vi "Create Config File Header.vi"(8 "error in (no error)":errorcluster, 10 "Path":path, 11 "Config Parser BML in":refnum<class "Config Parser BML.lvclass">) -> (0 "error out":errorcluster, 3 "Config Parser BML out":refnum<class "Config Parser BML.lvclass">)   [LabVIEW 2018, in "Config Parser BML.lvlib" / "Config Parser BML.lvclass"]
uses:
  Config Parser BML.lvclass
  <vilib>/Utility/file.llb/Write Delimited Spreadsheet (string).vi
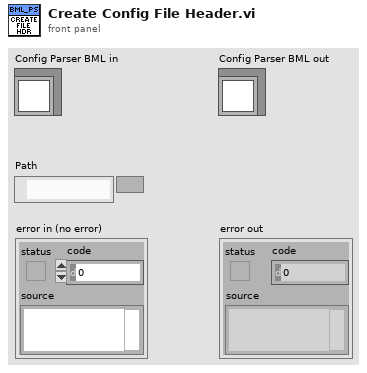
[diagram p1: front panel]
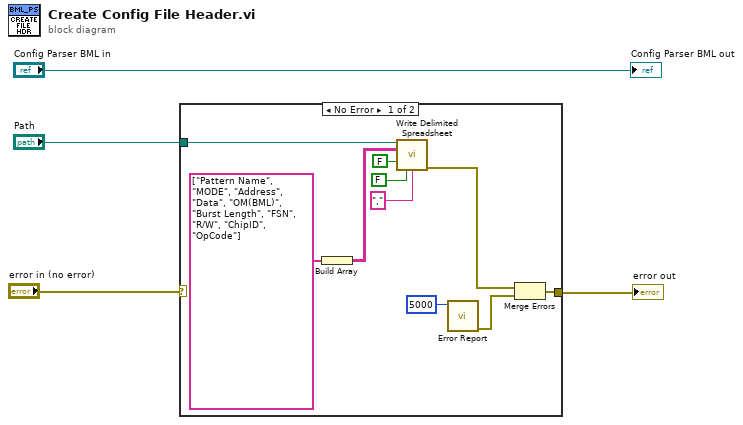
[diagram p0: block diagram]
diagram:
  n1 = case shown="No Error" "error in (no error)" {
    selector: "error in (no error)" -> [_ w15]
    tunnel: "Path" -> [w12 _]
    tunnel: [w7 w15] -> w1
    frame No Error {
      n2 = Build Array(string[] ["Pattern Name", "MODE", "Address", "Data", "OM(BML)", "Burst Length", "FSN", "R/W", "ChipID", "OpCode"]) -> (w10:string[][])
      n3 = call-poly <vilib>:"Write Delimited Spreadsheet.vi"("file path (dialog if empty)"=w12, "2D data"=w10, "append to file? (new file:F)"=FALSE, "transpose? (no:F)"=FALSE, "delimiter (\\t)"="," ("delimiter (\\t)")) -> ("error out"=w6:errorcluster)  [unwired: 9 in, 1 out]
      n4 = call "Error Report.vi"("Error Code"=i16 5000) -> ("error out"=w5:errorcluster)  [unwired: 10 in]
      n5 = Merge Errors(w6, w5) -> (w7:errorcluster)
    }
    frame Error {
    }
  }
  "error out" <- w1
  "Config Parser BML out" <- "Config Parser BML in"
